vi "Test API.vi"() -> ()   [LabVIEW 2015]
uses:
  Test Scope/Test Scope.lvclass
panel:
  out "JSON Data":string
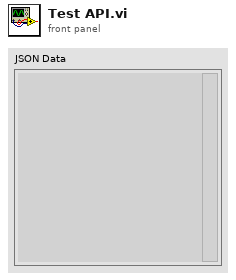
[diagram p1: front panel]
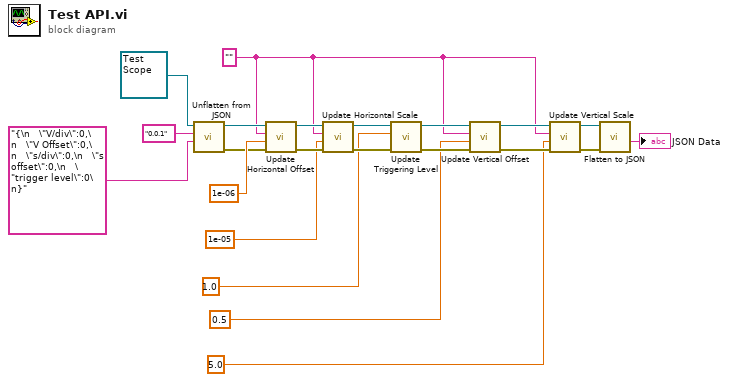
[diagram p0: block diagram]
diagram:
  w2 = "" ("Channel Name")
  n1 = call-dynamic "Unflatten from JSON.vi"("JSON Data"="{\n   \"V/div\":0,\n   \"V Offset\":0,\n   \"s/div\":0,\n   \"s offset\":0,\n   \"trigger level\":0\n}", "Version"="0.0.1", "Test Scope in"=refnum<class "Test Scope.lvclass"> refnum ("Test Scope.lvclass")) -> ("error out"=w6:errorcluster, "Test Scope out"=w7:refnum<class "Test Scope.lvclass">)  [unwired: 7 in]
  n2 = call-dynamic "Update Horizontal Offset.vi"("error in (no error)"=w6, "Offset (s)"=1e-06, "Channel Name"=w2, "Test Scope in"=w7) -> ("error out"=w21:errorcluster, "Test Scope out"=w22:refnum<class "Test Scope.lvclass">)  [unwired: 6 in]
  n3 = call-dynamic "Update Horizontal Scale.vi"("error in (no error)"=w21, "Seconds Per Division (s)"=1e-05, "Channel Name"=w2, "Test Scope in"=w22) -> ("error out"=w19:errorcluster, "Test Scope out"=w20:refnum<class "Test Scope.lvclass">)  [unwired: 6 in]
  n4 = call-dynamic "Update Triggering Level.vi"("error in (no error)"=w19, "Level (V)"=1.0, "Test Scope in"=w20) -> ("error out"=w17:errorcluster, "Test Scope out"=w18:refnum<class "Test Scope.lvclass">)  [unwired: 7 in]
  n5 = call-dynamic "Update Vertical Offset.vi"("error in (no error)"=w17, "Offset (V)"=0.5, "Channel Name"=w2, "Test Scope in"=w18) -> ("error out"=w15:errorcluster, "Test Scope out"=w16:refnum<class "Test Scope.lvclass">)  [unwired: 6 in]
  n6 = call-dynamic "Update Vertical Scale.vi"("error in (no error)"=w15, "Volts per Division (V)"=5.0, "Channel Name"=w2, "Test Scope in"=w16) -> ("error out"=w13:errorcluster, "Test Scope out"=w14:refnum<class "Test Scope.lvclass">)  [unwired: 6 in]
  n7 = call-dynamic "Flatten to JSON.vi"("error in (no error)"=w13, "Test Scope in"=w14) -> ("JSON Data"=→"JSON Data":string)  [unwired: 6 in, 3 out]
